vi "Ref Frame array-Build.vi"(0 "Single-frame buffer (in)":dbl[](array[numeric]), 1 "Logging queue element":T1={"Imaging Protocol"=enum."Live Imaging", "Number of Trials"=0, "Frame Size"=512, "# Averaged frames"=0, "Dwell time (us)"=0.0, "Index of Z-plane"=0, "Timelapse?"=FALSE, "Logging process is active"=FALSE, "Speed logging enabled"=FALSE, "tdms file ref"=refnum, "path"=path "", "Trial Number"=0, "Expected # points acquired"=FALSE, "Manually stopped"=FALSE, "Ch0 data"=[], "Ch1 data"=[], "Ref Data"=[], "Last trial"=FALSE, "Ref Dwell time (us)"=0.0, "# Ref Averaged frames"=0, "Ref X Length"=0, "Ref Y Length"=0, "Points acquired"={"Ch0 last trial"=0, "Ch1 last trial"=0, "All trials"=0}} {"Ref Dwell time (us)" format="%#.6g"; "Frame Size" items=["100X100"=100, "128X128"=128, "200X200"=200, "256X256"=256, "512X512"=512, "1024x1024"=1024, "2048x2048"=2048]; "Dwell time (us)" format="%#.6g"}, 9 "Number of points in single Ref frame buffer (in)":i32) -> (3 "Ref Frame Data":dbl[](array[numeric]), 4 "Single Ref frame buffer (out)":dbl[](array[numeric]), 6 "Ref frame completed/generate image":bool, 10 "Number of points in single Ref frame buffer":i32)   [LabVIEW 2017]
uses:
  Typedefs/Logging queue element.ctl
  Typedefs/Imaging Protocols enum.ctl
  Typedefs/Frame Size.ctl
  Typedefs/Acquired points count.ctl
panel:
  out "New chunk of scaled data (single channel)":dbl[](array[numeric])
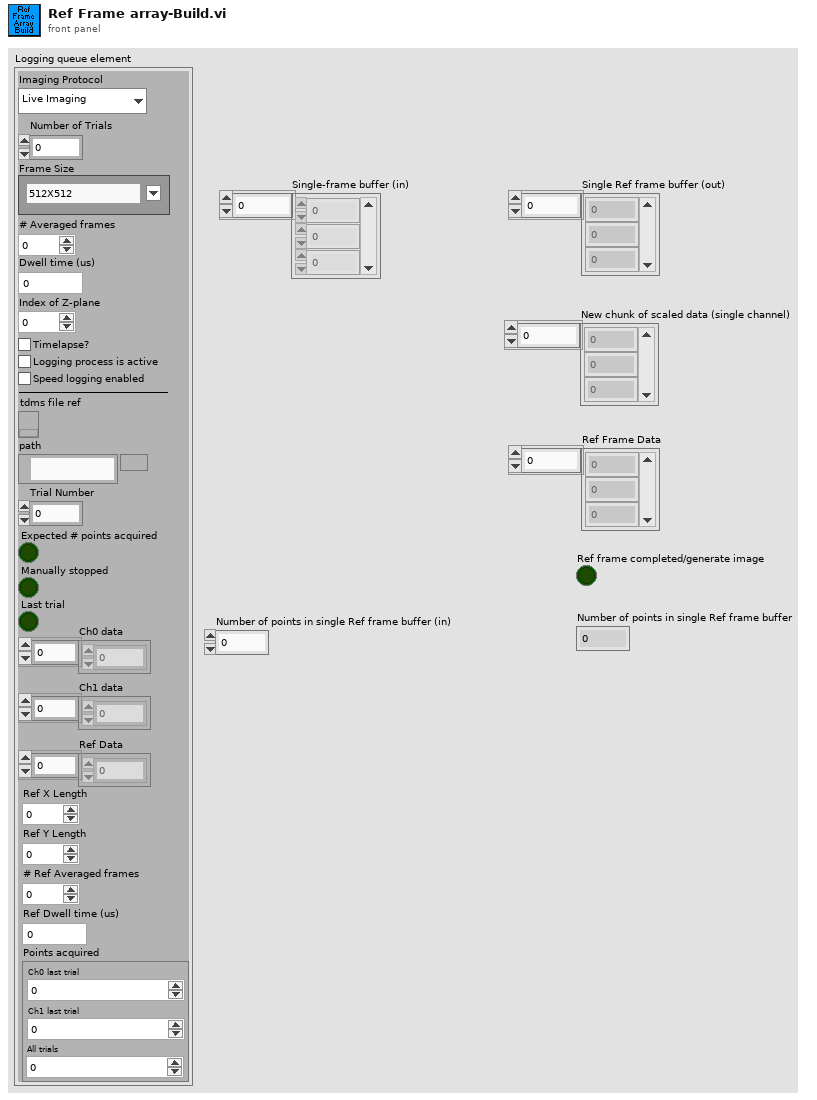
[diagram p1: front panel]
types:
  T1 = typedef "Logging queue element.ctl" = cluster{"Imaging Protocol":T2, "Number of Trials":u16, "Frame Size":T3, "# Averaged frames":u16, "Dwell time (us)":dbl, "Index of Z-plane":i32, "Timelapse?":bool, "Logging process is active":bool, "Speed logging enabled":bool, "tdms file ref":refnum<k34>, "path":path, "Trial Number":i32, "Expected # points acquired":bool, "Manually stopped":bool, "Ch0 data":u32[], "Ch1 data":u32[], "Ref Data":u32[], "Last trial":bool, "Ref Dwell time (us)":dbl, "# Ref Averaged frames":u16, "Ref X Length":u16, "Ref Y Length":u16, "Points acquired":T4}
  T2 = typedef "Imaging Protocols enum.ctl" = enum16{"AOL Z-Stack", "Motor Z Stack", "Functional Acquisition", "Single Plane Acquisition", "Volume Acquisition", "Live Imaging", "Live Plane Imaging", "Live Volume Imaging"}
  T3 = typedef "Frame Size.ctl" = u16
  T4 = typedef "Acquired points count.ctl" = cluster{"Ch0 last trial":u64, "Ch1 last trial":u64, "All trials":u64}
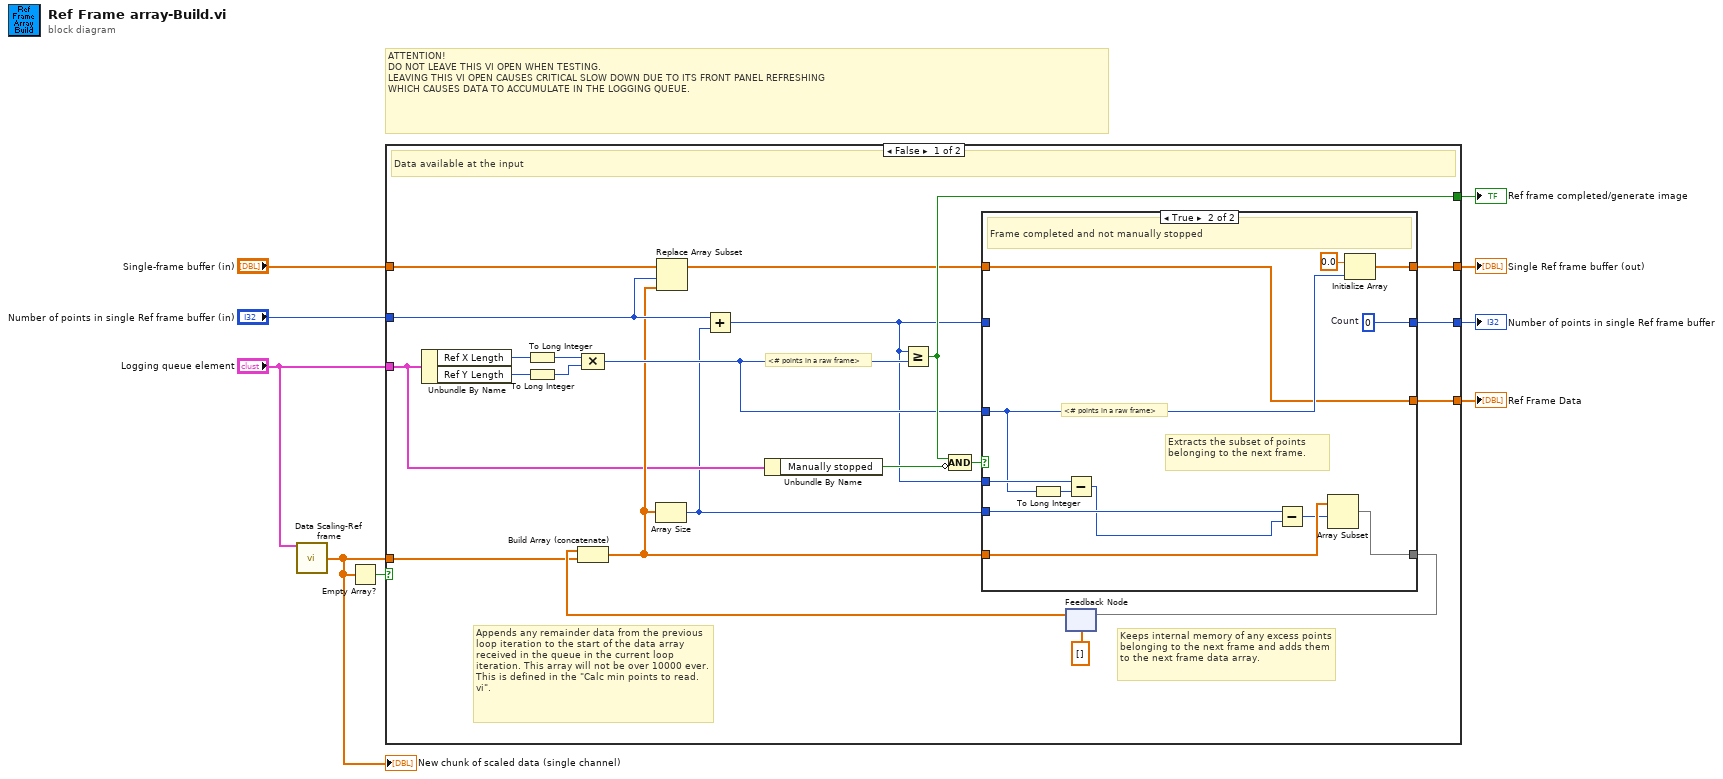
[diagram p0: block diagram]
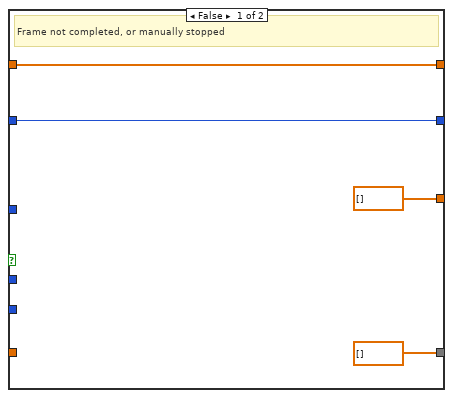
[diagram p2: hidden frame]
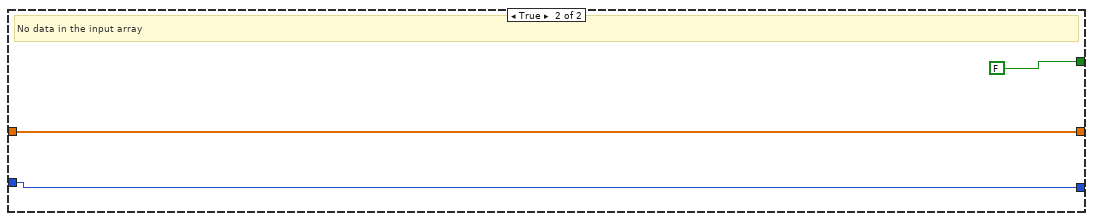
[diagram p3: hidden frame]
diagram:
  # "ATTENTION!\nDO NOT LEAVE THIS VI OPEN WHEN TESTING.\nLEAVING THIS VI OPEN CAUSES CRITICAL SLOW DOWN DUE TO ITS FRONT PANEL REFRESHING\nWHICH CAUSES DATA TO ACCUMULATE IN THE LOGGING QUEUE."
  n1 = call "Data Scaling-Ref frame.vi"("Logging queue element in"="Logging queue element") -> ("Scaled Ref data"=w1:dbl[])  [unwired: 13 in, 1 out]
  "New chunk of scaled data (single channel)" <- w1
  n2 = Empty Array?(array=w1) -> (empty?=w3:bool)
  n3 = case shown="False" w3 {
    tunnel: "Number of points in single Ref frame buffer (in)" -> [w31 w48]
    tunnel: [w30 FALSE] -> w8
    tunnel: "Single-frame buffer (in)" -> [w29 w49]
    tunnel: [w28 w48] -> w6
    tunnel: [w27 w49] -> w5
    tunnel: [w26 _] -> w4
    tunnel: "Logging queue element" -> [w17 _]
    tunnel: w1 -> [w16 _]
    frame False {
      # "<# points in a raw frame>"
      # "Appends any remainder data from the previous loop iteration to the start of the data array received in the queue in the current loop iteration. This array will not be over 10000 ever. This is defined in the \"Calc min points to read.vi\"."
      # "Keeps internal memory of any excess points belonging to the next frame and adds them to the next frame data array."
      # "Data available at the input"
      n4 = Unbundle By Name(w17) -> ("Ref X Length"=w24:u16, "Ref Y Length"=w15:u16)
      n5 = To Long Integer(number=w24) -> (32bit integer=w21:i32)
      n6 = To Long Integer(number=w15) -> (32bit integer=w14:i32)
      n7 = Compound Arithmetic op=MULTIPLY(w21, w14) -> (w20:i32)
      n8 = Unbundle By Name(w17) -> ("Manually stopped"=w22:bool)
      n9 = feedback #1(dbl[] []) -> (w19:dbl[])
      n10 = Build Array (concatenate)(w19, w16) -> (w18:dbl[])
      n11 = Array Size(array=w18) -> (size(s)=w12:i32)
      n12 = Replace Array Subset "Replace Array Subset"(array=w29, new element=w18, index=w31) -> (w10:dbl[])
      n13 = Add(x=w31, y=w12) -> (x+y=w11:i32)
      n14 = Greater Or Equal?(x=w11, y=w20) -> (x >= y?=w30:bool)
      n15 = Compound Arithmetic op=AND(w30, invert w22) -> (w13:bool)
      n16 = case shown="True" w13 {
        tunnel: w11 -> [_ w47]
        tunnel: w18 -> [_ w45]
        tunnel: w12 -> [_ w46]
        tunnel: [dbl[] [] w44] -> w25
        tunnel: w10 -> [w33 w36]
        tunnel: w11 -> [w34 _]
        tunnel: [w34 w41] -> w28
        tunnel: [w33 w42] -> w27
        tunnel: w20 -> [_ w37]
        tunnel: [dbl[] [] w36] -> w26
        frame False {
          # "Frame not completed, or manually stopped"
        }
        frame True {
          w41 = 0  # Count
          # "<# points in a raw frame>"
          # "Extracts the subset of points belonging to the next frame."
          # "Frame completed and not manually stopped"
          n17 = To Long Integer(number=w37) -> (32bit integer=w40:i32)
          n18 = Subtract(x=w47, y=w40) -> (x-y=w39:i32)
          n19 = Subtract(x=w46, y=w39) -> (x-y=w38:i32)
          n20 = Array Subset "Array Subset"(array=w45, index=w38) -> (w44:dbl[])  [unwired: 1 in]
          n21 = Initialize Array(0.0, w37) -> (w42:dbl[])
        }
      }
      n22 = feedback-in #1(w25) -> ()
    }
    frame True {
      # "No data in the input array"
    }
  }
  "Number of points in single Ref frame buffer" <- w6
  "Single Ref frame buffer (out)" <- w5
  "Ref frame completed/generate image" <- w8
  "Ref Frame Data" <- w4
